vi "Analog Knob.vi"() -> ()   [LabVIEW 2016]
uses:
  <vilib>/rvi/Emulation/niFpgaGetClockAttributes.vi
  <vilib>/rvi/Emulation/niFpgaSctlEmulationGetInTimedLoop.vi
  <vilib>/rvi/Emulation/niFpgaEmulationReportErrorSimple.vi
  <vilib>/rvi/eio/common/nirviEmuTemplateMethod_errors.vi
  <vilib>/rvi/Emulation/niFpgaCriticalErrorInLSC.vi
  <vilib>/eio/EIONode/EIONode.xnode
panel:
  out "Boolean":bool
  in  "stop":bool
  out "Waveform Chart":sgl(graph)
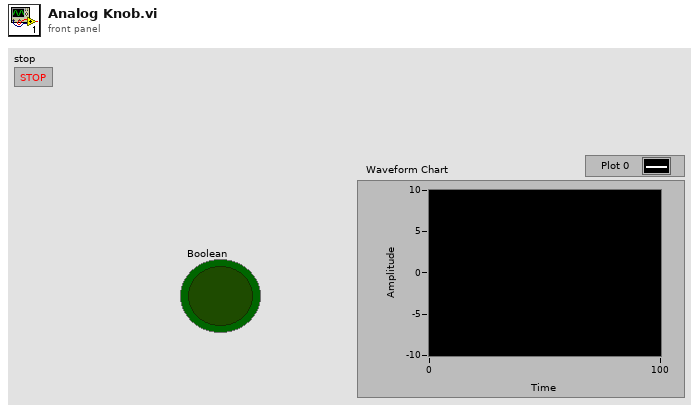
[diagram p1: front panel]
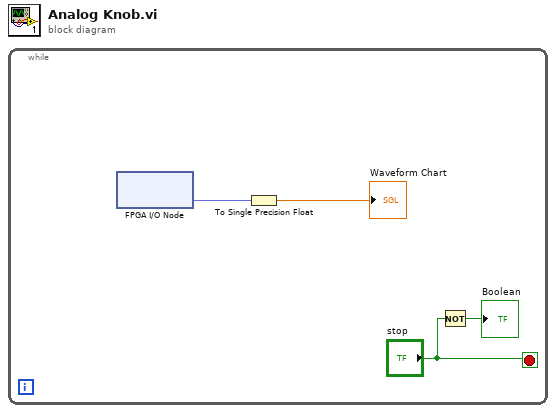
[diagram p0: block diagram]
diagram:
  n1 = while {
    stop <- "stop" stop-if-true
    n2 = xnode "FPGA I/O Node"() -> ("AI6"=w4:fxp<+/-,24,5>)  [unwired: 1 in, 1 out]
    n3 = To Single Precision Float(number=w4) -> (single precision float=→"Waveform Chart":sgl)
    n4 = Not(x="stop") -> (.not. x?=→"Boolean":bool)
  }
